vi "9-2.vi"() -> (3 "Numeric":i32)   [LabVIEW 2022 SP3, in "AoC22.lvlib"]
uses:
  AoC22.lvlib
  <vilib>/Utility/miscctls.llb/LVMapReplaceAction.ctl
  <vilib>/IlluminatedG/lv-stream/Stream.lvlib
panel:
  out "Head":cluster{"Row":i32, "Col":i32}
  out "Tail":cluster{"Row":i32, "Col":i32}
  in  "OK Button":bool
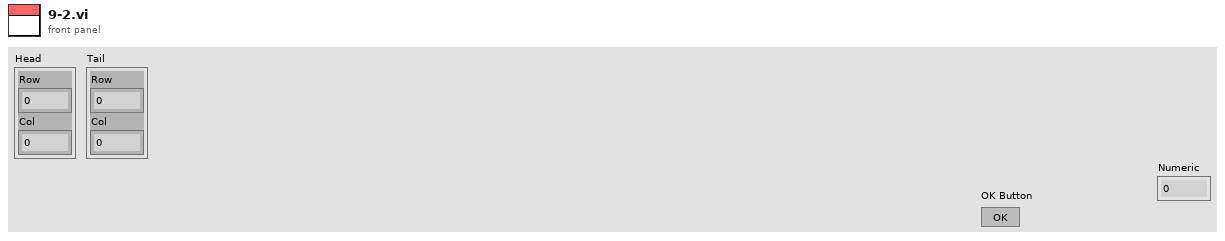
[diagram p1: front panel]
types:
  T1 = map{cluster{"Row":i32, "Col":i32}, cluster{"Tail Count":i32}}
  T2 = typedef "LVMapReplaceAction.ctl" = enum32{"Modify Entry only if found", "Add or Modify Entry", "Delete Entry"}
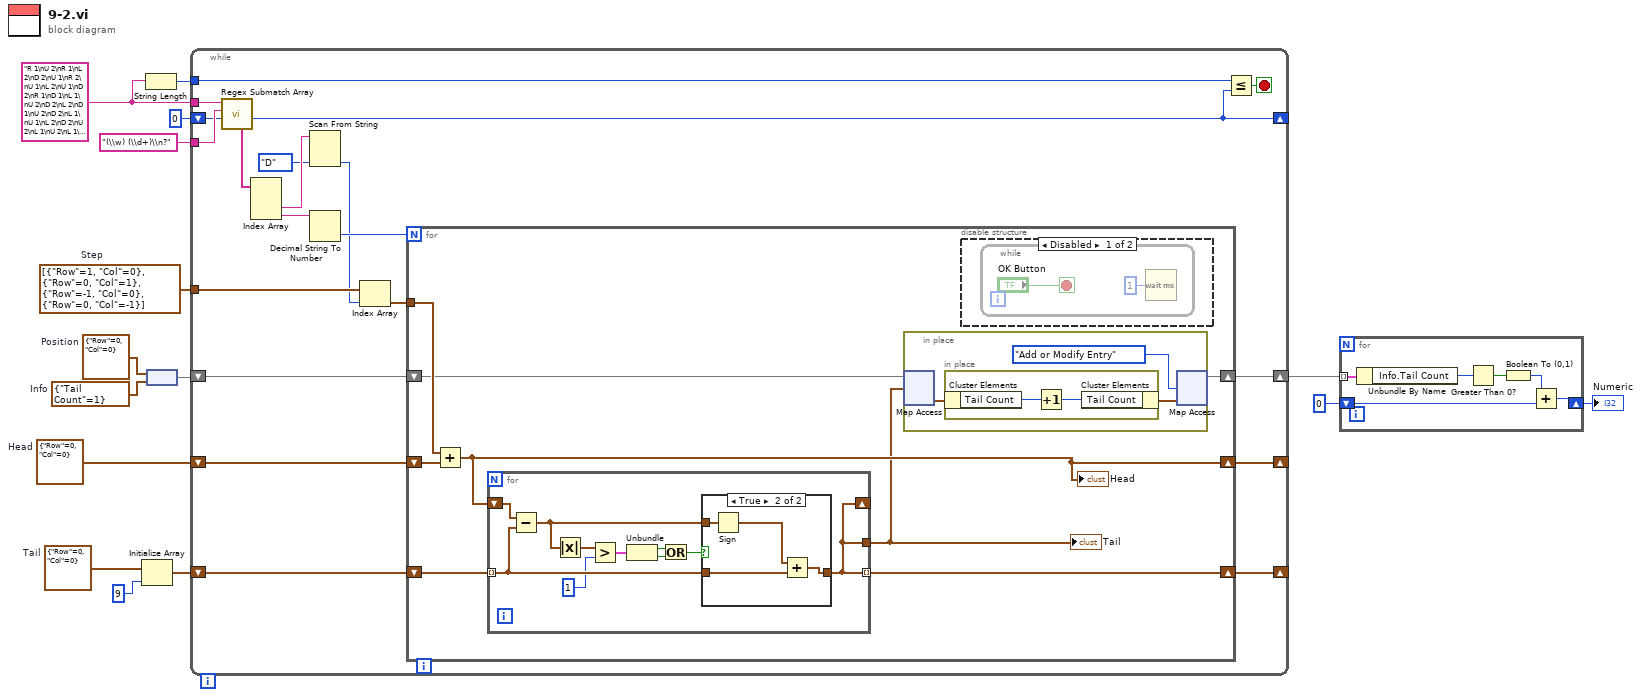
[diagram p0: block diagram]
diagram:
  w8 = cluster{"Tail Count":i32} {"Tail Count"=1}  # Info
  w10 = cluster{"Row":i32, "Col":i32} {"Row"=0, "Col"=0}  # Position
  w11 = cluster{"Row":i32, "Col":i32}[] [{"Row"=1, "Col"=0}, {"Row"=0, "Col"=1}, {"Row"=-1, "Col"=0}, {"Row"=0, "Col"=-1}]  # Step
  w2 = cluster{"Row":i32, "Col":i32} {"Row"=0, "Col"=0}  # Tail
  w3 = cluster{"Row":i32, "Col":i32} {"Row"=0, "Col"=0}  # Head
  w13 = "R 1\nU 2\nR 1\nL 2\nD 2\nU 1\nR 2\nU 1\nL 2\nU 1\nD 2\nR 1\nD 1\nL 1\nU 2\nD 2\nL 2\nD 1\nU 2\nD 2\nL 1\nU 1\nL 2\nD 2\nU 2\nL 1\nU 2\nL 1\nR 2\nU 1\nL 1\nR 2\nD 1\nU 2\nR 1\nU 1\nR 2\nU 1\nR 2\nU 1\nD 1\nU 1\nD 1\nL 2\nD 2\nR 1\nU 1\nR 1\nU 1\nL 1\nU 1\nD 2\nR 2\nD 2\nL 2\nU 2\nR 1\nD 1\nU 1\nD 2\nR 1\nD 2\nL 2\nR 2\nL 1\nU 1\nL 2\nD 2\nL 2\nD 1\nR 1\nL 2\nD 2\nR 1\nL 1\nR 1\nD 1\nR 1\nD 2\nL 2\nU 1\nD 2\nR 2\nD 1\nU 1\nL 1\nD 1\nU 2\nR 1\nU 1\nL 2\nU 1\nL 1\nU 2\nL 2\nD 2\nU 1\nL 1\nU 2\nD 2\nL 2\nD 2\nR 2\nU 2\nL 2\nD 1\nU 1\nR 2\nD 2\nL 2\nR 2\nD 2\nL 1\nD 1\nU 2\nR 2\nD 3\nR 1\nU 3\nL 3\nD 2\nR 1\nD 1\nL 2\nD 1\nR 2\nU 3\nL 2\nU 2\nR 3\nU 3\nL 1\nD 3\nR 3\nU 2\nR 3\nU 3\nL 1\nD 3\nR 3\nL 2\nR 2\nL 3\nD 3\nR 2\nD 2\nR 2\nD 1\nR 1\nL 1\nD 2\nR 1\nD 2\nU 1\nR 2\nL 2\nR 2\nU 2\nR 2\nD 1\nU 1\nD 1\nL 3\nU 3\nD 3\nL 1\nU 2\nR 2\nU 2\nR 1\nU 1\nL 2\nU 2\nR 3\nU 1\nD 3\nR 3\nU 2\nR 1\nU 1\nD 3\nL 2\nU 3\nL 1\nR 2\nD 3\nR 2\nU 1\nR 2\nD 1\nU 3\nL 2\nD 1\nR 1\nL 3\nR 3\nD 2\nR 1\nU 2\nR 3\nD 2\nU 2\nL 2\nU 1\nR 2\nU 2\nL 2\nD 3\nL 2\nD 1\nL 1\nU 2\nL 1\nD 2\nR 1\nD 2\nR 1\nL 2\nU 1\nL 1\nU 1\nD 2\nR 4\nD 4\nL 2\nR 4\nD 1\nL 2\nD 2\nL 4\nU 4\nD 4\nL 3\nR 3\nD 1\nL 1\nD 1\nU 4\nR 4\nU 4\nD 2\nR 1\nU 3\nR 2\nU 3\nR 4\nD 3\nU 3\nL 4\nD 1\nR 2\nU 3\nD 4\nU 3\nR 2\nL 1\nD 2\nU 2\nR 3\nU 2\nR 2\nD 2\nL 2\nU 4\nR 1\nL 3\nR 1\nL 1\nD 3\nR 4\nD 2\nR 4\nU 3\nL 1\nD 1\nR 4\nU 3\nD 1\nL 3\nR 1\nL 3\nD 2\nL 2\nR 3\nL 4\nD 4\nU 1\nL 1\nR 1\nD 3\nL 2\nR 1\nD 3\nR 2\nD 4\nU 4\nR 3\nU 1\nD 3\nL 3\nD 3\nU 1\nD 2\nU 4\nR 4\nU 2\nD 1\nR 1\nD 4\nL 2\nR 3\nU 4\nL 1\nD 1\nU 4\nL 3\nD 4\nU 2\nR 4\nU 2\nR 4\nU 2\nL 1\nR 1\nL 3\nD 4\nL 2\nR 2\nL 3\nU 3\nR 4\nL 2\nR 1\nD 5\nU 1\nR 1\nU 2\nR 1\nU 4\nL 3\nU 4\nR 2\nD 3\nL 4\nR 3\nL 2\nU 2\nR 1\nL 3\nD 5\nR 3\nL 2\nU 5\nR 2\nU 5\nL 5\nU 4\nR 4\nD 2\nR 4\nD 3\nR 2\nD 3\nU 2\nL 3\nD 3\nL 1\nU 4\nD 3\nL 1\nD 1\nR 2\nL 4\nR 3\nU 1\nR 3\nL 2\nR 3\nD 4\nR 2\nU 3\nL 4\nR 5\nL 1\nU 1\nD 5\nU 2\nR 5\nL 4\nD 3\nL 1\nD 3\nU 1\nR 2\nD 1\nL 5\nD 2\nR 4\nL 1\nD 2\nR 4\nL 3\nR 3\nL 3\nR 4\nL 3\nU 3\nD 4\nU 2\nR 1\nD 1\nU 1\nR 5\nD 5\nL 5\nR 3\nU 2\nD 4\nL 5\nD 1\nL 4\nR 4\nU 2\nL 2\nR 2\nU 3\nL 1\nU 3\nL 1\nD 4\nU 5\nD 5\nR 4\nL 4\nR 5\nD 4\nU 5\nL 4\nU 1\nD 4\nR 5\nD 2\nU 4\nR 2\nU 3\nD 2\nU 6\nD 4\nR 1\nD 4\nR 3\nL 1\nR 5\nU 6\nD 5\nL 4\nR 3\nL 4\nR 5\nD 1\nR 3\nD 2\nL 6\nU 5\nR 6\nL 2\nD 6\nU 1\nL 3\nD 4\nR 6\nD 3\nL 3\nR 5\nU 6\nD 5\nU 1\nR 4\nL 4\nU 4\nR 5\nD 1\nL 4\nU 6\nL 2\nR 3\nL 2\nR 3\nL 3\nR 4\nU 3\nD 1\nR 6\nD 5\nL 2\nR 4\nU 4\nD 2\nL 1\nR 2\nD 3\nL 4\nD 4\nR 4\nD 6\nR 1\nL 2\nR 5\nD 3\nU 5\nR 4\nL 6\nD 6\nU 4\nR 4\nL 4\nU 4\nR 5\nD 1\nU 1\nR 4\nL 2\nU 6\nD 3\nL 3\nU 6\nD 1\nU 4\nD 6\nR 6\nU 1\nR 2\nU 5\nD 4\nL 2\nU 5\nD 1\nL 5\nU 1\nR 3\nD 2\nR 1\nL 3\nD 1\nR 1\nL 2\nR 6\nD 6\nR 4\nU 4\nL 5\nR 6\nL 5\nR 4\nD 3\nL 2\nR 4\nL 2\nU 6\nD 5\nR 1\nL 3\nR 1\nU 2\nR 6\nL 2\nD 7\nL 2\nD 4\nR 2\nU 6\nD 4\nR 5\nU 6\nR 3\nL 3\nU 2\nR 3\nU 1\nR 7\nU 2\nR 2\nD 7\nR 1\nU 5\nD 1\nL 5\nU 5\nR 2\nD 5\nR 4\nU 5\nL 3\nD 4\nL 6\nR 7\nL 2\nD 3\nL 2\nD 6\nU 6\nL 1\nD 7\nU 6\nL 7\nR 5\nL 1\nU 7\nR 1\nL 4\nR 4\nL 5\nU 7\nD 4\nR 7\nL 5\nU 7\nL 6\nU 3\nD 5\nR 5\nU 7\nR 5\nL 3\nU 6\nR 2\nU 3\nR 3\nU 6\nL 5\nD 6\nL 4\nD 5\nR 1\nL 3\nU 6\nR 6\nU 6\nL 1\nD 2\nL 5\nD 1\nL 6\nU 5\nD 5\nR 5\nD 6\nL 4\nU 5\nR 2\nU 4\nD 7\nL 1\nU 1\nD 1\nL 1\nD 4\nU 1\nL 6\nU 1\nR 5\nD 1\nU 1\nR 1\nU 5\nR 4\nU 5\nL 2\nU 6\nL 7\nR 2\nU 4\nR 5\nL 1\nR 8\nL 2\nD 7\nR 7\nD 2\nL 2\nR 2\nD 2\nU 7\nD 7\nR 4\nU 1\nR 2\nL 6\nU 1\nL 3\nU 2\nD 7\nR 6\nL 5\nD 1\nL 3\nU 6\nD 2\nU 2\nR 4\nD 1\nL 7\nU 3\nD 8\nU 4\nD 8\nL 8\nU 6\nL 3\nU 4\nR 4\nU 8\nD 1\nR 7\nU 5\nL 8\nU 4\nL 4\nD 7\nU 8\nL 2\nD 8\nL 1\nR 1\nL 1\nR 8\nL 8\nR 5\nL 1\nR 4\nD 3\nR 2\nU 8\nL 6\nR 4\nL 3\nR 8\nL 4\nD 5\nR 3\nU 2\nD 8\nU 4\nR 6\nD 4\nR 3\nL 7\nD 8\nL 2\nU 6\nD 7\nR 3\nL 5\nR 4\nD 3\nL 4\nR 8\nL 7\nD 8\nR 3\nU 3\nL 3\nR 6\nL 1\nU 3\nL 1\nU 4\nR 8\nL 8\nR 2\nD 3\nL 2\nR 1\nD 2\nR 6\nU 3\nD 1\nU 3\nR 1\nU 2\nR 2\nL 2\nD 6\nU 7\nL 8\nD 6\nU 2\nR 3\nL 6\nU 9\nD 6\nU 1\nD 3\nU 4\nR 3\nL 9\nD 6\nU 9\nD 1\nL 5\nU 5\nD 6\nU 4\nL 8\nU 8\nD 3\nL 3\nU 9\nR 5\nL 7\nD 1\nR 9\nU 8\nD 1\nR 1\nU 9\nD 4\nR 6\nU 8\nR 6\nU 3\nD 2\nU 8\nL 8\nU 9\nD 4\nL 3\nU 4\nD 3\nL 9\nR 7\nL 9\nR 3\nL 5\nD 7\nL 8\nU 9\nL 7\nD 1\nL 6\nU 7\nL 6\nD 8\nU 9\nL 7\nR 7\nD 1\nR 6\nD 4\nU 7\nR 7\nL 8\nD 4\nR 1\nL 7\nD 2\nU 3\nD 1\nR 7\nD 7\nR 7\nL 6\nD 9\nU 7\nD 5\nR 7\nL 1\nR 9\nU 1\nL 2\nU 5\nR 4\nD 7\nR 2\nD 5\nU 4\nD 3\nR 9\nU 2\nD 9\nU 1\nR 9\nU 9\nD 1\nL 7\nU 6\nD 6\nU 9\nL 5\nU 2\nD 6\nL 4\nD 3\nU 1\nR 2\nL 1\nR 1\nD 1\nR 1\nU 1\nR 4\nL 7\nR 2\nD 1\nU 3\nD 3\nR 10\nL 7\nR 7\nD 2\nL 6\nR 9\nU 9\nD 8\nU 9\nR 2\nU 6\nD 9\nU 1\nL 2\nR 10\nL 9\nR 10\nL 6\nR 4\nD 4\nR 4\nU 4\nD 4\nL 5\nR 8\nD 4\nL 7\nD 6\nL 8\nR 9\nL 8\nD 7\nR 2\nU 2\nD 5\nL 4\nR 8\nD 7\nR 6\nD 7\nL 5\nU 7\nR 1\nD 7\nR 9\nD 5\nU 3\nL 8\nD 7\nU 4\nD 4\nR 10\nU 7\nD 4\nU 2\nR 7\nL 4\nU 2\nD 9\nL 5\nR 2\nU 10\nL 9\nR 10\nL 1\nD 5\nR 10\nL 5\nR 5\nD 5\nR 10\nL 4\nU 9\nD 7\nR 10\nL 6\nU 3\nD 5\nU 6\nL 6\nU 10\nL 1\nU 10\nD 4\nL 7\nU 2\nL 10\nR 4\nL 7\nR 4\nD 10\nL 4\nU 10\nL 10\nD 9\nU 4\nR 8\nU 8\nR 5\nU 3\nD 10\nR 7\nL 10\nR 9\nL 1\nD 6\nL 11\nD 11\nR 3\nL 8\nU 6\nR 9\nD 5\nR 9\nD 4\nU 7\nD 4\nR 4\nU 10\nD 4\nR 2\nL 3\nU 5\nD 11\nR 8\nL 8\nU 7\nR 3\nD 8\nU 5\nR 10\nD 5\nR 2\nU 11\nD 10\nR 1\nU 9\nL 10\nR 2\nD 11\nR 6\nL 3\nR 10\nU 2\nD 6\nL 10\nU 5\nL 6\nU 1\nR 10\nU 8\nR 8\nD 4\nU 8\nL 11\nR 7\nL 2\nD 2\nR 5\nU 10\nL 3\nR 6\nL 8\nR 8\nU 8\nD 3\nL 7\nR 5\nL 6\nD 11\nL 6\nD 7\nU 6\nD 3\nU 9\nL 7\nR 8\nL 3\nR 10\nD 11\nL 11\nR 4\nD 6\nL 7\nD 9\nR 10\nU 11\nL 9\nD 8\nL 2\nU 1\nD 7\nU 10\nD 11\nR 5\nD 11\nL 6\nD 5\nR 6\nD 5\nR 11\nU 3\nD 6\nR 5\nU 7\nD 2\nR 6\nU 5\nD 9\nU 3\nR 7\nD 10\nU 5\nD 4\nR 6\nU 11\nL 10\nU 5\nL 6\nR 5\nU 7\nL 7\nR 5\nD 9\nU 11\nL 7\nU 8\nL 7\nU 3\nL 8\nR 10\nU 11\nR 8\nL 12\nU 8\nD 2\nL 2\nD 2\nU 10\nR 11\nU 2\nR 6\nU 3\nD 9\nU 5\nD 12\nL 11\nD 8\nU 12\nR 4\nU 1\nL 2\nR 10\nD 6\nL 10\nU 2\nR 4\nL 4\nD 8\nU 9\nL 4\nD 10\nU 5\nR 10\nL 2\nD 2\nU 2\nR 7\nD 8\nR 1\nU 11\nD 1\nL 7\nR 12\nD 12\nR 3\nL 11\nR 10\nU 11\nR 5\nD 6\nR 11\nD 2\nL 3\nD 12\nL 9\nR 6\nU 1\nD 2\nR 6\nD 5\nU 7\nR 2\nD 5\nU 3\nD 12\nR 12\nL 9\nR 9\nD 12\nR 8\nD 11\nL 7\nU 4\nD 11\nR 1\nU 9\nL 1\nD 2\nR 3\nU 1\nD 1\nR 2\nD 11\nU 12\nR 7\nD 1\nU 13\nL 5\nD 13\nL 10\nD 12\nL 7\nD 9\nL 7\nU 6\nL 1\nR 1\nL 10\nR 7\nL 6\nU 7\nR 10\nU 7\nR 11\nU 12\nL 2\nD 11\nL 5\nU 2\nD 8\nL 10\nD 13\nU 10\nL 9\nU 5\nD 11\nR 6\nL 9\nR 2\nL 6\nU 4\nR 7\nD 11\nL 3\nU 6\nD 13\nU 2\nR 13\nU 11\nL 12\nD 13\nL 1\nR 9\nD 10\nU 6\nL 13\nU 2\nL 12\nD 7\nR 1\nL 6\nD 1\nU 10\nD 5\nL 2\nU 12\nR 1\nU 9\nD 4\nU 10\nL 1\nR 1\nU 8\nR 2\nD 1\nL 6\nU 11\nD 2\nU 7\nD 11\nU 9\nD 6\nU 5\nD 13\nR 2\nU 8\nL 4\nU 4\nR 2\nU 1\nD 3\nL 1\nD 13\nR 9\nL 4\nD 5\nL 7\nU 2\nD 10\nL 6\nU 11\nD 1\nU 5\nR 4\nD 9\nR 12\nD 2\nU 9\nL 10\nU 6\nD 2\nL 8\nU 4\nL 4\nD 12\nU 3\nL 14\nD 12\nR 12\nL 7\nU 5\nL 2\nD 4\nL 13\nD 10\nL 8\nD 12\nR 13\nU 8\nD 14\nU 4\nR 11\nL 4\nR 13\nL 2\nU 1\nD 10\nL 12\nD 13\nL 4\nD 11\nR 14\nU 8\nL 11\nD 2\nU 8\nL 8\nD 3\nL 14\nU 7\nL 2\nR 2\nD 6\nU 1\nL 12\nR 12\nU 4\nL 1\nU 13\nR 12\nD 8\nU 10\nR 2\nL 7\nR 4\nD 4\nL 14\nU 2\nD 2\nU 11\nL 7\nR 12\nU 9\nL 11\nR 6\nD 6\nR 8\nL 1\nD 9\nL 7\nD 10\nR 6\nD 6\nL 5\nD 14\nL 12\nU 12\nR 4\nD 14\nL 10\nD 11\nL 3\nD 3\nU 9\nL 6\nD 10\nU 1\nL 10\nD 9\nR 8\nL 3\nU 7\nR 4\nU 9\nL 5\nR 7\nD 7\nL 5\nU 4\nR 4\nL 7\nR 8\nL 2\nR 5\nL 10\nR 2\nL 12\nD 12\nL 6\nR 4\nL 11\nD 13\nL 13\nR 10\nD 12\nU 5\nR 11\nL 15\nR 6\nU 9\nD 5\nU 6\nL 1\nD 1\nR 7\nD 5\nR 15\nU 11\nR 5\nD 15\nR 13\nU 8\nR 11\nU 7\nD 4\nL 6\nD 11\nU 1\nL 2\nR 11\nL 12\nD 5\nR 3\nL 14\nR 15\nL 14\nU 13\nD 9\nL 3\nD 4\nU 9\nL 3\nR 14\nU 3\nR 15\nL 14\nR 4\nU 15\nL 1\nD 11\nL 13\nD 14\nL 1\nD 1\nU 13\nD 7\nU 13\nD 15\nU 15\nL 6\nD 7\nR 15\nL 10\nU 6\nR 7\nL 13\nU 3\nD 9\nL 3\nD 10\nR 14\nD 15\nL 6\nD 4\nU 11\nL 11\nD 6\nU 8\nD 15\nR 5\nL 9\nD 15\nU 15\nR 9\nD 11\nU 7\nL 9\nU 8\nD 2\nL 4\nD 11\nU 12\nR 11\nU 5\nL 12\nU 5\nR 14\nL 10\nR 6\nD 3\nL 13\nU 6\nR 10\nD 10\nU 9\nD 3\nR 7\nL 13\nR 15\nU 6\nL 13\nU 11\nD 9\nL 7\nR 8\nU 6\nR 12\nU 2\nL 8\nU 10\nD 11\nU 14\nR 3\nL 15\nU 9\nL 2\nU 2\nD 11\nL 11\nR 3\nD 14\nU 3\nL 1\nU 2\nD 12\nL 5\nR 5\nD 10\nL 16\nR 4\nU 3\nL 6\nR 9\nL 7\nR 2\nU 15\nR 6\nL 12\nD 16\nL 16\nD 15\nU 12\nL 6\nD 9\nU 8\nL 10\nD 11\nU 4\nD 12\nU 7\nD 14\nU 1\nD 10\nR 10\nD 14\nL 5\nD 6\nR 8\nL 16\nU 7\nL 12\nR 13\nL 11\nD 12\nR 5\nD 11\nL 5\nR 4\nD 15\nL 13\nD 10\nR 2\nL 16\nD 14\nR 15\nD 11\nU 2\nD 12\nL 11\nD 1\nR 5\nD 6\nU 13\nL 10\nR 1\nU 10\nD 12\nL 10\nD 10\nR 11\nL 10\nD 11\nL 3\nR 11\nD 12\nL 6\nU 2\nL 10\nD 9\nL 11\nU 12\nD 14\nL 6\nU 16\nD 2\nL 2\nD 14\nU 7\nR 12\nD 14\nL 4\nU 3\nR 16\nD 2\nL 5\nR 10\nL 1\nR 11\nL 14\nD 3\nL 17\nD 4\nU 1\nR 8\nD 8\nL 5\nU 1\nL 13\nD 15\nU 17\nL 1\nD 14\nU 4\nR 1\nU 2\nD 14\nR 10\nU 14\nD 17\nR 10\nU 13\nD 12\nU 8\nL 11\nU 17\nR 12\nU 6\nD 8\nR 10\nU 16\nD 4\nR 3\nD 3\nU 4\nL 3\nU 5\nR 16\nL 5\nR 16\nD 17\nR 12\nL 11\nR 13\nU 12\nL 8\nR 5\nD 6\nU 16\nL 16\nD 2\nL 11\nD 1\nR 1\nD 14\nR 15\nL 6\nU 14\nR 12\nD 11\nL 9\nU 6\nL 11\nD 15\nU 17\nL 1\nU 3\nL 6\nU 5\nR 16\nL 14\nR 9\nL 12\nD 14\nU 13\nL 3\nU 13\nD 7\nR 2\nU 7\nD 5\nL 17\nD 6\nL 16\nR 5\nD 4\nR 3\nU 11\nD 3\nU 9\nD 10\nU 2\nL 6\nD 6\nR 15\nD 17\nR 1\nL 15\nD 2\nU 5\nR 2\nD 6\nL 8\nR 5\nL 2\nD 17\nU 9\nD 9\nL 7\nR 12\nL 12\nR 18\nL 10\nR 9\nD 6\nR 9\nU 15\nL 17\nD 18\nR 1\nL 15\nD 4\nR 6\nU 3\nR 6\nU 3\nD 1\nU 9\nD 8\nR 3\nD 6\nU 3\nR 8\nL 8\nR 10\nU 7\nD 16\nU 17\nR 11\nU 8\nD 1\nU 8\nL 4\nR 12\nD 10\nU 7\nD 18\nU 7\nD 12\nL 18\nU 9\nR 2\nU 5\nD 14\nR 13\nD 15\nU 17\nD 16\nL 4\nD 10\nL 2\nU 7\nL 7\nD 13\nR 13\nU 12\nR 16\nU 17\nR 3\nU 12\nR 6\nD 12\nU 11\nL 6\nU 15\nL 12\nR 1\nD 6\nL 16\nR 1\nD 7\nR 17\nL 15\nD 15\nU 9\nR 18\nD 13\nR 14\nD 1\nR 1\nD 16\nL 18\nR 1\nU 14\nL 8\nD 14\nR 15\nD 2\nU 10\nD 17\nU 3\nD 9\nR 7\nD 17\nU 3\nD 15\nL 17\nD 17\nR 1\nD 10\nL 9\nD 14\nR 5\nU 14\nR 14\nD 12\nR 18\nU 4\nD 2\nU 17\nD 12\nL 4\nU 9\nL 9\nU 17\nR 4\nU 17\nR 8\nD 10\nR 3\nD 9\nU 17\nL 5\nR 16\nU 9\nL 5\nD 15\nU 2\nD 7\nL 15\nU 1\nL 16\nR 8\nL 13\nR 3\nD 8\nR 1\nD 8\nL 10\nU 16\nR 16\nL 2\nU 3\nD 9\nU 12\nD 1\nL 10\nD 15\nU 7\nR 3\nD 15\nU 4\nL 6\nR 14\nU 13\nR 16\nU 2\nR 9\nU 15\nD 8\nL 8\nR 17\nD 3\nL 17\nD 13\nU 8\nD 11\nR 13\nL 3\nD 2\nU 14\nR 1\nU 10\nR 11\nD 16\nL 10\nR 17\nU 7\nL 13\nR 3\nL 18\nR 5\nU 7\nL 12\nD 4\nU 5\nL 17\nR 18\nL 4\nR 19\nL 12\nU 17\nR 2\nL 11\nR 9\nD 16\nR 19\nL 18\nU 11\nD 4\nR 13\nL 18\nU 13\nR 19\nD 3\nR 10\nL 3\nR 5\nD 2\nR 2\nL 18\nD 15\nR 19\nL 5\nD 4\nU 5\nR 12\nD 15\nL 13\nR 16\nU 16\nL 6\nU 12\nL 8"
  n1 = Initialize Array(w2, 9 ("dimension size")) -> (w1:cluster{"Row":i32, "Col":i32}[])
  n2 = String Length(string=w13) -> (length=w12:i32)
  n3 = node(w10, w8) -> (w9:T1)
  n4 = while {
    tunnel: w13 -> [w35]
    tunnel: "(\\w) (\\d+)\\n?" ("regular expression") -> [w30]
    shift-right: [w17] -> _
    shift-left: w3 -> [w21]
    shift-right: [w16] -> _
    shift-left: w1 -> [w20]
    shift-right: [w27] -> _
    shift-left: 0 ("offset past match") -> [w29]
    tunnel: w12 -> [w28]
    shift-right: [w18] -> w7
    shift-left: w9 -> [w19]
    tunnel: w11 -> [w24]
    stop <- w26 stop-if-true
    n5 = call <vilib>:"Regex Submatch Array.vi"("offset (0)"=w29, "regular expression"=w30, "string"=w35) -> ("offset past match"=w27:i32, "matches"=w34:string[])  [unwired: 6 in, 1 out]
    n6 = Index Array(array=w34) -> (element #2=w32:string, element #3=w33:string)  [unwired: 3 in, 1 out]
    n7 = Scan From String(input string=w32, default 1=enum16{"U", "R", "D", "L"}."D") -> (output 1=w23:enum16{"U", "R", "D", "L"})  [unwired: 3 in, 3 out]
    n8 = Decimal String To Number(string=w33) -> (number=w25:i32)  [unwired: 2 in, 1 out]
    n9 = Index Array(array=w24, index=w23) -> (element=w22:cluster{"Row":i32, "Col":i32})
    n10 = for {
      N: w25 -> [_]
      shift-right: [w41] -> w17
      shift-left: w21 -> [w43]
      shift-right: [w37] -> w16
      shift-left: w20 -> [w40]
      tunnel: w22 -> [w42]
      shift-right: [w39] -> w18
      shift-left: w19 -> [w38]
      n11 = Add(x=w42, y=w43) -> (x+y=w41:cluster{"Row":i32, "Col":i32})
      "Head" <- w41
      n12 = for {
        tunnel: w40 -> [w52] mode=indexing
        tunnel: [w44] -> w37 mode=indexing
        tunnel: [w44] -> w36
        shift-right: [w44] -> _
        shift-left: w41 -> [w53]
        n13 = Subtract(x=w53, y=w52) -> (x-y=w51:cluster{"Row":i32, "Col":i32})
        n14 = Absolute Value(x=w51) -> (abs(x)=w50:cluster{"Row":i32, "Col":i32})
        n15 = Greater?(x=w50, y=1) -> (0:w46:cluster{"Row":bool, "Col":bool})
        n16 = Unbundle(w46) -> ("Row"=w47:bool, "Col"=w48:bool)
        n17 = Or(x=w47, y=w48) -> (x .or. y?=w45:bool)
        n18 = case shown="True" w45 {
          tunnel: w52 -> [w54 w57]
          tunnel: w51 -> [_ w58]
          tunnel: [w54 w55] -> w44
          frame False {
          }
          frame True {
            n19 = Sign(1:w58) -> (0:w56:cluster{"Row":i32, "Col":i32})
            n20 = Add(x=w56, y=w57) -> (x+y=w55:cluster{"Row":i32, "Col":i32})
          }
        }
      }
      "Tail" <- w36
      n21 = in-place {
        n22 = in-place-map #1(w38, w36) -> (w62:cluster{"Tail Count":i32})  [unwired: 1 in, 1 out]
        n23 = in-place {
          n24 = in-place-cluster #2(w62) -> ("Tail Count"=w65:i32)
          n25 = Increment(x=w65) -> (x+1=w64:i32)
          n26 = in-place-cluster #2("Tail Count"=w64) -> (w61:cluster{"Tail Count":i32})
        }
        n27 = in-place-map #1(w61, LVMapReplaceAction."Add or Modify Entry" ("action")) -> (w39:T1)  [unwired: 2 out]
      }
      n28 = disable-structure shown="Disabled" {
        frame Disabled {
          n29 = while {
            stop <- "OK Button" stop-if-true
            n30 = Wait (ms)(milliseconds to wait=u32 1) -> ()  [unwired: 1 out]
          }
        }
        frame Enabled {
        }
      }
    }
    n31 = Less Or Equal?(x=w28, y=w27) -> (x <= y?=w26:bool)
  }
  n32 = for {
    tunnel: w7 -> [w71] mode=indexing
    shift-right: [w66] -> w5
    shift-left: 0 -> [w67]
    n33 = Unbundle By Name(w71) -> ("Info.Tail Count"=w70:i32)
    n34 = Greater Than 0?(x=w70) -> (x > 0?=w69:bool)
    n35 = Boolean To (0,1)(Boolean=w69) -> (0, 1=w68:i16)
    n36 = Add(x=w68, y=w67) -> (x+y=w66:i32)
  }
  "Numeric" <- w5
